vi "SDO Download_.vi"(6 "Value":variant, 7 "Sync?":bool, 8 "error in":errorcluster, 9 "Multiplexor":T1 {"Sub-Index" format="%.0x"; "Index" format="%.0x"}, 10 "Node ID":u8, 11 "CANopen in":refnum<class "CANopen.lvclass">) -> (0 "error out":errorcluster, 3 "CANopen out":refnum<class "CANopen.lvclass">)   [LabVIEW 2024, in "canopen.lvlib" / "CANopen.lvclass"]
doc: "Writes a value in the open dictionary of a CANopen node."
uses:
  CANopen.lvclass
  CANopen.lvclass/CANopen.ctl
  Multiplexer.ctl
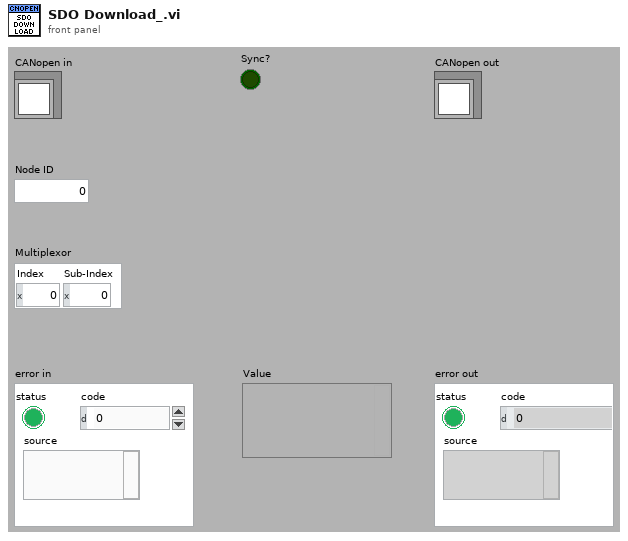
[diagram p1: front panel]
types:
  T1 = typedef "canopen.lvlib/CANopen.lvclass/Multiplexer.ctl" = cluster{"Index":u16, "Sub-Index":u8}
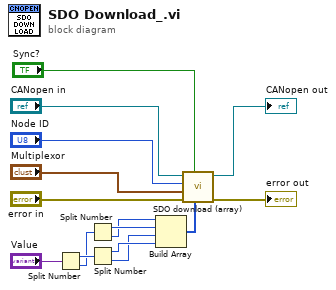
[diagram p0: block diagram]
diagram:
  n1 = Split Number(x="Value") -> (hi(x)=w4:u16, lo(x)=w3:u16)
  n2 = Split Number(x=w3) -> (hi(x)=w8:u8, lo(x)=w7:u8)
  n3 = Split Number(x=w4) -> (hi(x)=w6:u8, lo(x)=w5:u8)
  n4 = Build Array(w7, w8, w5, w6) -> (w10:u8[])
  n5 = call "SDO download (array).vi"("Value"=w10, "Wait?"="Sync?", "error in"="error in", "Multiplexor"="Multiplexor", "Node ID"="Node ID", "CANopen in"="CANopen in") -> ("error out"=→"error out":errorcluster, "CANopen out"=→"CANopen out":refnum<class "CANopen.lvclass">)  [unwired: 4 in]
